vi "Process.vi"(8 "error in":errorcluster, 11 "Qbus in":refnum<class "Qbus.lvclass">) -> (0 "error out":errorcluster)   [LabVIEW 2021, in "EventLoggerProcess.lvlib"]
uses:
  EventLoggerProcess.lvlib
  <vilib>/addons/Qbus/Qbus.lvclass
  controls/event.ctl
  <vilib>/NI/Event Logger Library/EventLog/Initialize_CSV.vi
  <vilib>/NI/Event Logger Library/EventLog/EventLog.lvclass
  generation/subVIs/utility/AudioGenUtility.lvlib
  <vilib>/NI/LogRotate/LogRotate.lvclass
  <vilib>/NI/LogRotate/options.ctl
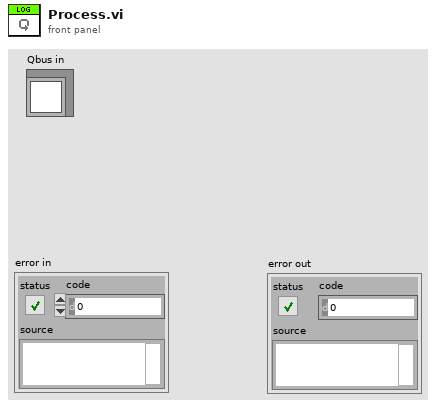
[diagram p1: front panel]
types:
  T1 = typedef "LogRotate.lvclass/options.ctl" = cluster{"max file size (bytes)":i64, "rotate count":u32, "max age (days)":dbl, "No archive dir":bool, "Archive dir":path}
  T2 = typedef "EventLoggerProcess.lvlib/event.ctl" = cluster{"name":string, "description":string}
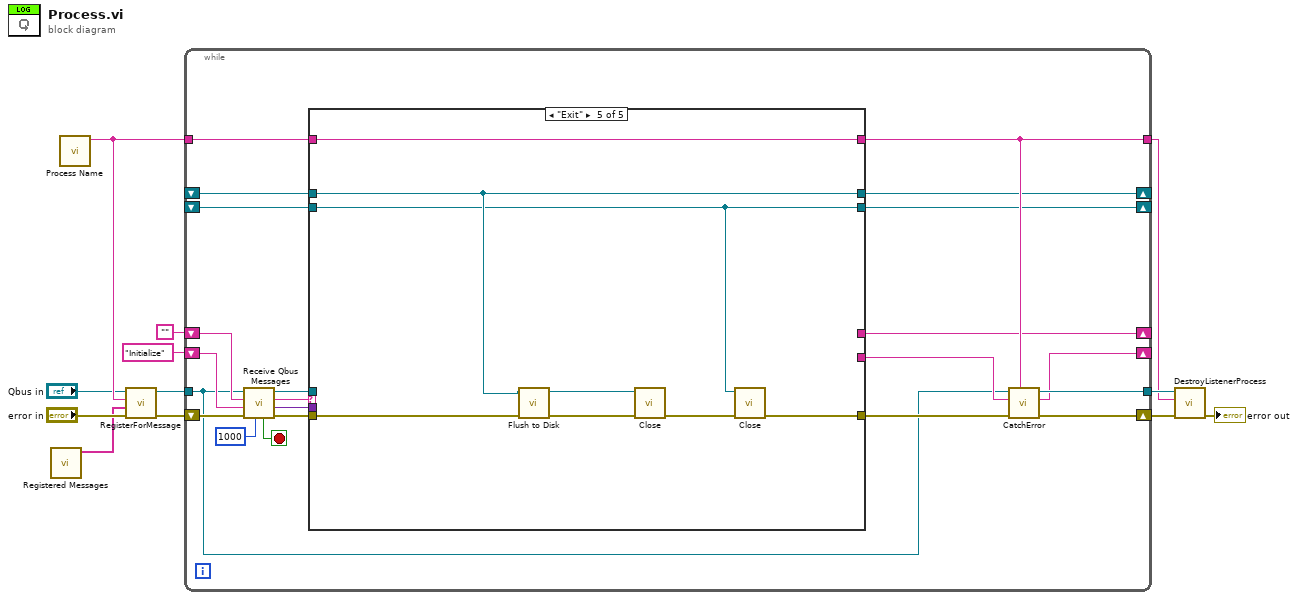
[diagram p0: block diagram]
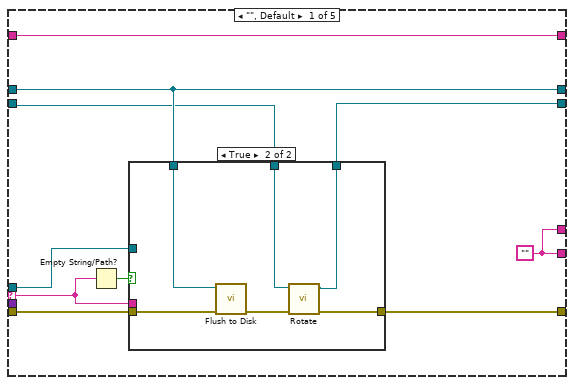
[diagram p2: hidden frame]
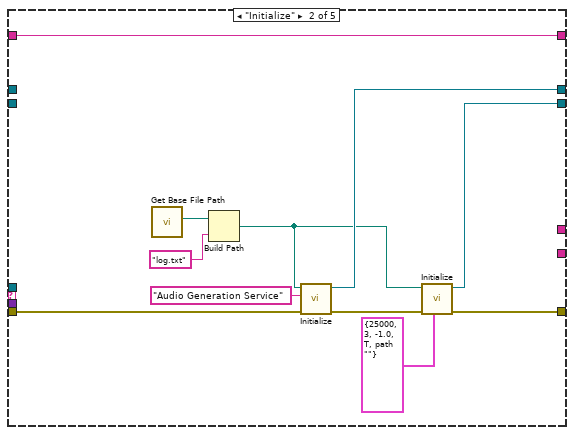
[diagram p4: hidden frame]
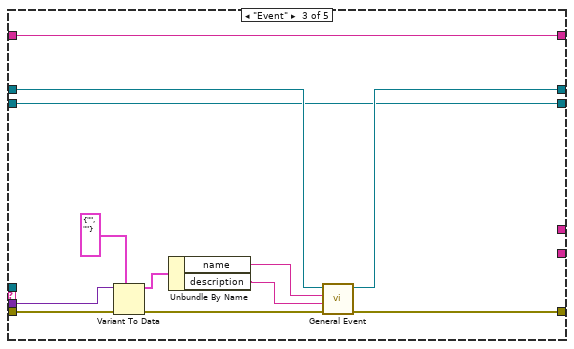
[diagram p5: hidden frame]
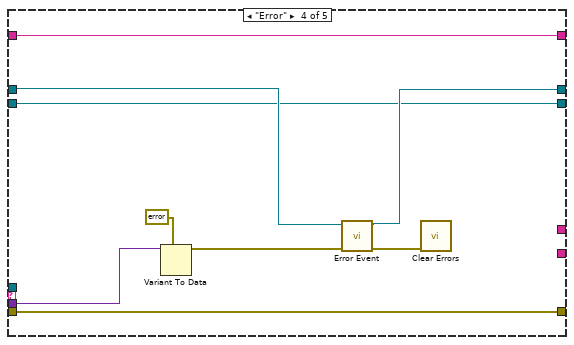
[diagram p6: hidden frame]
diagram:
  n1 = call "Registered Messages.vi"() -> ("registered messages"=w5:string[])  [unwired: 11 in]
  n2 = call "Process Name.vi"() -> ("process name"=w8:string)  [unwired: 11 in]
  n3 = call <vilib>:"RegisterForMessage.vi"("error in (no error)"="error in", "message names"=w5, "process name"=w8, "Qbus in"="Qbus in") -> ("error in (no error)"=w11:errorcluster, "Qbus out"=w12:refnum<class "Qbus.lvclass">)  [unwired: 6 in]
  n4 = while {
    shift-right: [w20] -> _
    shift-left: "" -> [w33]
    tunnel: w12 -> [w18]
    tunnel: w8 -> [w17]
    tunnel: [w27] -> w3
    tunnel: [w22] -> w1
    shift-right: [w26] -> _
    shift-left: "Initialize" -> [w29]
    shift-right: [w28] -> w4
    shift-left: w11 -> [w25]
    shift-right: [w16] -> _
    shift-left: _ -> [w15]
    shift-right: [w14] -> _
    shift-left: _ -> [w13]
    stop <- w34 stop-if-true
    n5 = call "Receive Qbus Messages.vi"("timeout(ms)"=1000 ("milliseconds to wait"), "error in (no error)"=w25, "priority action"=w29, "default action"=w33, "Qbus in"=w18) -> ("error out"=w32:errorcluster, "message value"=w30:variant, "action"=w24:string, "Qbus out"=w31:refnum<class "Qbus.lvclass">, "exit"=w34:bool)  [unwired: 2 in]
    n6 = case shown="\"Exit\"" w24 {
      selector: w24 -> [w41 _ _ _ _]
      tunnel: w32 -> [w43 w62 w71 w84 w91]
      tunnel: w31 -> [w39 _ _ _ _]
      tunnel: [w42 w54 w74 w84 w85] -> w19
      tunnel: w30 -> [_ _ w68 w80 _]
      tunnel: [w44 w63 w75 w83 w92] -> w22
      tunnel: w17 -> [w44 w63 w75 w83 w92]
      tunnel: [w38 _ _ _ _] -> w21
      tunnel: [w38 _ _ _ _] -> w20
      tunnel: [w37 w61 w72 w81 w88] -> w16
      tunnel: w15 -> [w37 _ w73 w82 w88]
      tunnel: [w35 w55 w64 w76 w86] -> w14
      tunnel: w13 -> [w36 _ w64 w76 w86]
      frame "", Default {
        w38 = ""
        n7 = Empty String/Path?(string/path=w41) -> (empty?=w40:bool)
        n8 = case shown="True" w40 {
          tunnel: [w46 w49] -> w42
          tunnel: w43 -> [w46 w52]
          tunnel: w41 -> [_ _]
          tunnel: w39 -> [_ _]
          tunnel: w37 -> [_ w51]
          tunnel: w36 -> [w45 w48]
          tunnel: [w45 w47] -> w35
          frame False {
          }
          frame True {
            n9 = call <vilib>:"Flush to Disk.vi"("error in (no error)"=w52, "EventLog ref"=w51) -> ("error out"=w50:errorcluster)  [unwired: 8 in, 1 out]
            n10 = call <vilib>:"Rotate.vi"("error in (no error)"=w50, "LogRotate in"=w48) -> ("error out"=w49:errorcluster, "LogRotate out"=w47:refnum<class "LogRotate.lvclass">)  [unwired: 8 in]
          }
        }
      }
      frame "Initialize" {
        n11 = call "Get Base File Path.vi"() -> ("base path"=w59:path)  [unwired: 11 in]
        n12 = Build Path(base path=w59, name or relative path="log.txt") -> (appended path=w56:path)
        n13 = call-poly <vilib>:"Initialize.vi"("error in (no error)"=w62, "Description"="Audio Generation Service", "Path"=w56) -> ("error out"=w57:errorcluster, "EventLog ref"=w61:refnum<class "EventLog.lvclass">)  [unwired: 7 in]
        n14 = call <vilib>:"Initialize.vi"("Options"=T1 {"max file size (bytes)"=25000, "rotate count"=3, "max age (days)"=-1.0, "No archive dir"=TRUE, "Archive dir"=path ""}, "error in (no error)"=w57, "Log File Path"=w56) -> ("error out"=w54:errorcluster, "LogRotate"=w55:refnum<class "LogRotate.lvclass">)  [unwired: 7 in]
      }
      frame "Event" {
        n15 = Variant To Data(error in=w71, type=T2 {"name"="", "description"=""} ("event"), Variant=w68) -> (data=w67:T2, error out=w70:errorcluster)
        n16 = Unbundle By Name(w67) -> ("name"=w66:string, "description"=w65:string)
        n17 = call <vilib>:"General Event.vi"("error in (no error)"=w70, "Event Description"=w65, "Event Name"=w66, "EventLog ref"=w73) -> ("error out"=w74:errorcluster, "EventLog ref"=w72:refnum<class "EventLog.lvclass">)  [unwired: 6 in]
      }
      frame "Error" {
        n18 = Variant To Data(type=errorcluster {"status"=FALSE, "code"=0, "source"=""} ("error in (no error)"), Variant=w80) -> (data=w78:errorcluster)  [unwired: 1 in, 1 out]
        n19 = call <vilib>:"Error Event.vi"("error in (no error)"=w78, "EventLog ref"=w82) -> ("error out"=w77:errorcluster, "EventLog ref"=w81:refnum<class "EventLog.lvclass">)  [unwired: 8 in]
        n20 = call <vilib>:"Clear Errors.vi"("error in (no error)"=w77) -> ()  [unwired: 5 in, 2 out]
      }
      frame "Exit" {
        n21 = call <vilib>:"Flush to Disk.vi"("error in (no error)"=w91, "EventLog ref"=w88) -> ("error out"=w90:errorcluster, "EventLog ref"=w89:refnum<class "EventLog.lvclass">)  [unwired: 8 in]
        n22 = call <vilib>:"Close.vi"("error in (no error)"=w90, "EventLog ref"=w89) -> ("error out"=w87:errorcluster)  [unwired: 9 in]
        n23 = call <vilib>:"Close.vi"("error in (no error)"=w87, "LogRotate"=w86) -> ("error out"=w85:errorcluster)  [unwired: 9 in]
      }
    }
    n24 = call <vilib>:"CatchError.vi"("source"=w22, "error in (no error)"=w19, "next action in"=w21, "Qbus in"=w18) -> ("error out"=w28:errorcluster, "next action out"=w26:string, "Qbus out"=w27:refnum<class "Qbus.lvclass">)  [unwired: 5 in]
  }
  n25 = call <vilib>:"DestroyListenerProcess.vi"("error in (no error)"=w4, "process name"=w1, "Qbus in"=w3) -> ("error in (no error)"=→"error out":errorcluster)  [unwired: 7 in, 1 out]
